vi "RegenerateFilesMetadata.vi"(8 "error in (no error)":errorcluster, 10 "Path":path, 11 "head in":refnum<data-value>) -> (0 "error out":errorcluster, 2 "String":string, 3 "head out":refnum<data-value>)   [LabVIEW 2017]
uses:
  DirectoryMetadata/DirectoryMetadata.lvclass
  PathConfiguration.vi
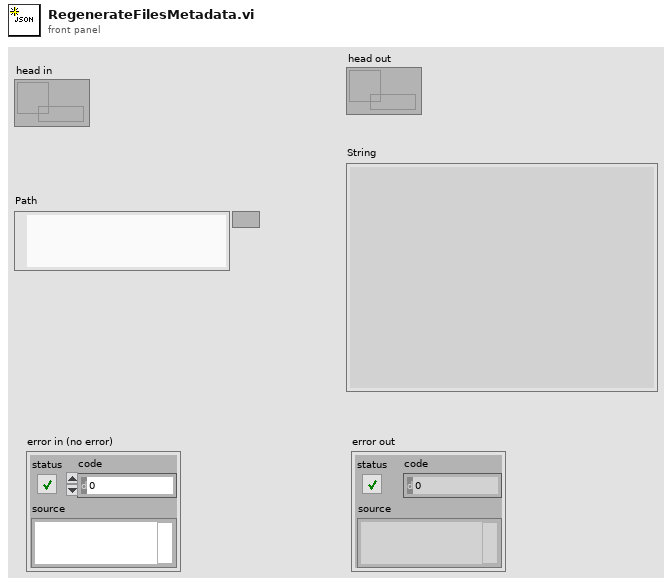
[diagram p1: front panel]
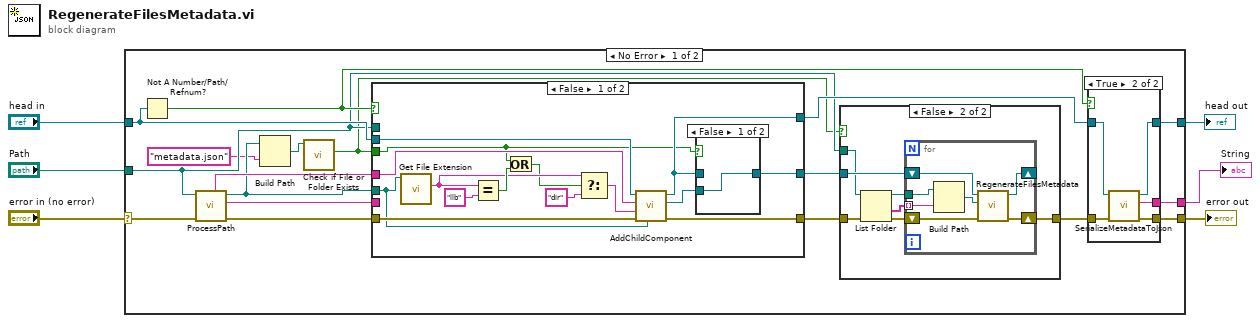
[diagram p0: block diagram]
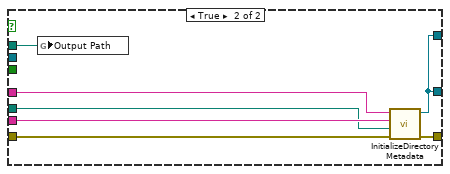
[diagram p4: hidden frame]
diagram:
  n1 = case shown="No Error" "error in (no error)" {
    selector: "error in (no error)" -> [w20 w72]
    tunnel: "Path" -> [w10 _]
    tunnel: "head in" -> [w19 w71]
    tunnel: [w16 w72] -> w5
    tunnel: [w18 w71] -> w4
    tunnel: [w15 _] -> w3
    frame No Error {
      n2 = Not A Number/Path/Refnum?(number/path/refnum=w19) -> (NaN/Path/Refnum?=w11:bool)
      n3 = call "ProcessPath.vi"("error in (no error)"=w20, "path in"=w10) -> ("error out"=w13:errorcluster, "Type"=w24:string, "path out"=w12:path, "File/Folder name"=w23:string)  [unwired: 5 in, 1 out]
      n4 = Build Path(base path=w12, name or relative path="metadata.json") -> (appended path=w9:path)
      n5 = call <vilib>:"Check if File or Folder Exists.vi"("path"=w9) -> ("file or folder exists?"=w7:bool)  [unwired: 8 in, 2 out]
      n6 = case shown="False" w11 {
        tunnel: w13 -> [w45 w55]
        tunnel: w24 -> [_ w54]
        tunnel: w23 -> [w43 w53]
        tunnel: [w42 w51] -> w22
        tunnel: [w44 w52] -> w21
        tunnel: w19 -> [w46 _]
        tunnel: [w40 w51] -> w14
        tunnel: w12 -> [w38 w50]
        tunnel: w10 -> [_ w49]
        tunnel: w7 -> [w36 _]
        frame False {
          n7 = call <vilib>:"Get File Extension.vi"("file"=w38) -> ("lowercase file extension"=w34:string)  [unwired: 6 in, 4 out]
          n8 = Equal?(x=w34, y="llb") -> (x = y?=w35:bool)
          n9 = Or(x=w36, y=w35) -> (x .or. y?=w32:bool)
          n10 = Select(t=w34, s=w32, f="dir" ("File/Folder name")) -> (s? t:f=w37:string)
          n11 = call "AddChildComponent.vi"("Path"=w38, "error in (no error)"=w45, "Type"=w37, "ID"=w43, "head in"=w46) -> ("error out"=w44:errorcluster, "child ref"=w41:refnum<data-value>, "head out"=w40:refnum<data-value>)  [unwired: 4 in]
          n12 = case shown="False" w36 {
            tunnel: [w47 w48] -> w42
            tunnel: w41 -> [w47 _]
            tunnel: w40 -> [_ w48]
            frame False {
            }
            frame True {
            }
          }
        }
        frame True {
          n13 = global write "PathConfiguration.vi" "Output Path"(w49) -> ()
          n14 = call "InitializeDirectoryMetadata.vi"("Error in"=w55, "Path"=w50, "Type"=w54, "ID"=w53) -> ("Error out"=w52:errorcluster, "DirectoryMetadata instance"=w51:refnum<data-value>)  [unwired: 6 in]
        }
      }
      n15 = case shown="False" w7 {
        tunnel: w21 -> [w56 w63]
        tunnel: w10 -> [_ w59]
        tunnel: [w56 w61] -> w17
        tunnel: w22 -> [_ w60]
        frame True {
        }
        frame False {
          n16 = List Folder(path=w59, error in=w63) -> (path out=w58:path, folder names=w57:string[], error out=w62:errorcluster)  [unwired: 2 in, 1 out]
          n17 = for {
            shift-right: [w67] -> w61
            shift-left: w62 -> [w68]
            shift-right: [w69] -> _
            shift-left: w60 -> [w70]
            tunnel: w58 -> [w66]
            tunnel: w57 -> [w65] mode=indexing
            n18 = Build Path(base path=w66, name or relative path=w65) -> (appended path=w64:path)
            n19 = call "RegenerateFilesMetadata.vi"("error in (no error)"=w68, "Path"=w64, "head in"=w70) -> ("error out"=w67:errorcluster, "head out"=w69:refnum<data-value>)  [unwired: 6 in, 1 out]
          }
        }
      }
      n20 = case shown="True" w11 {
        tunnel: [w25 w31] -> w18
        tunnel: w17 -> [w26 w30]
        tunnel: [w26 w29] -> w16
        tunnel: [_ w28] -> w15
        tunnel: w14 -> [w25 w27]
        frame False {
        }
        frame True {
          n21 = call "SerializeMetadataToJson.vi"("error in (no error)"=w30, "head in"=w27) -> ("error out"=w29:errorcluster, "Serialized String"=w28:string, "head out"=w31:refnum<data-value>)  [unwired: 7 in]
        }
      }
    }
    frame Error {
    }
  }
  "error out" <- w5
  "head out" <- w4
  "String" <- w3
